vi "CreateSEQ.vi"() -> (3 "FPGA out":refnum<queue>, 5 "created new?":bool)   [LabVIEW 2019, in "FPGA.lvlib"]
uses:
  FPGA.lvlib
  FPGA.ctl
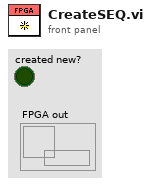
[diagram p1: front panel]
types:
  T1 = typedef "FPGA.lvlib/FPGA.ctl" = cluster{"Start freq. [Hz]":dbl, "Sweep duration [s]":dbl, "Freq. step [Hz]":dbl, "DAC Sample Rate":dbl, "ADC Sample Rate":dbl, "CMD port":u16, "DFAST port":u16, "CMD ID":refnum<k16>, "DFAST ID":refnum<k16>, "CMD error out":errorcluster, "FPGA IP":string, "DFAST error out ":errorcluster, "Stop freq. [Hz]":dbl, "Discrete sweep":bool, "Initial NCO":u32, "Difference NCO":i32, "step NCO":i64, "Final NCO":u32, "clocks for step":u32, "demodulation":bool, "NCO Phase Precision":u32, "NCO Sample Rate":dbl, "Time for step [s]":dbl, "NCO freq. resolution":dbl, "Sweep speed [Hz/s]":dbl, "Connected":bool, "Slew Rate [V/us]":dbl, "Parameters_ok":bool, "Amplitude [mVpp]":dbl, "Scale Factor":fxp<+,16,0>, "Acquiring":bool, "DAC-ADC Latency":u16, "Digital Gain":i32, "Number of steps":i32, "Averaging preferred":bool, "Filter Order":u32, "Settling":enum16{"99%", "99,9%"}}
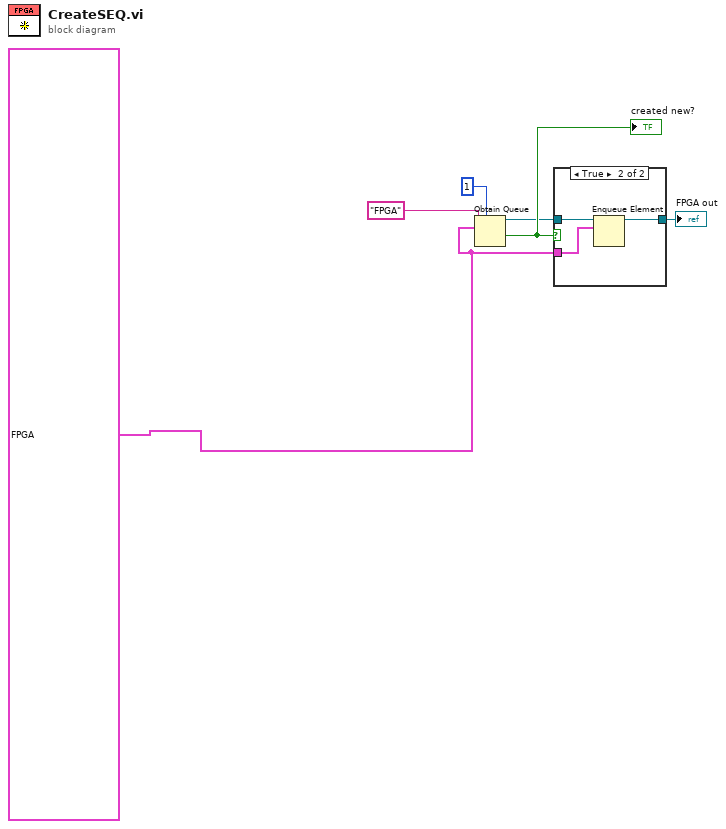
[diagram p0: block diagram]
diagram:
  w1 = T1 {"Start freq. [Hz]"=10.0, "Sweep duration [s]"=0.1, "Freq. step [Hz]"=0.1, "DAC Sample Rate"=1388888.8888, "ADC Sample Rate"=50000000.0, "CMD port"=2047, "DFAST port"=2048, "CMD ID"=refnum, "DFAST ID"=refnum, "CMD error out"={"status"=FALSE, "code"=0, "source"=""}, "FPGA IP"="192.168.1.12", "DFAST error out "={"status"=FALSE, "code"=0, "source"=""}, "Stop freq. [Hz]"=0.0, "Discrete sweep"=FALSE, "Initial NCO"=10, "Difference NCO"=0, "step NCO"=0, "Final NCO"=0, "clocks for step"=0, "demodulation"=FALSE, "NCO Phase Precision"=32, "NCO Sample Rate"=50000000.0, "Time for step [s]"=0.1, "NCO freq. resolution"=32.0, "Sweep speed [Hz/s]"=0.1, "Connected"=FALSE, "Slew Rate [V/us]"=0.8, "Parameters_ok"=FALSE, "Amplitude [mVpp]"=10.0, "Scale Factor"=0.999969482421875, "Acquiring"=FALSE, "DAC-ADC Latency"=1, "Digital Gain"=0, "Number of steps"=1, "Averaging preferred"=FALSE, "Filter Order"=1, "Settling"=enum."99,9%"} ("FPGA CLUSTER")
  n1 = Obtain Queue(max queue size (-1, unlimited)=1, name (unnamed)="FPGA" ("FPGA Name"), element data type=w1) -> (queue out=w5:refnum<queue>, created new?=w6:bool)  [unwired: 2 in, 1 out]
  "created new?" <- w6
  n2 = case shown="True" w6 {
    tunnel: w5 -> [w7 w10]
    tunnel: w1 -> [_ w9]
    tunnel: [w7 w8] -> w2
    frame False {
    }
    frame True {
      n3 = Enqueue Element(queue=w10, element=w9) -> (queue out=w8:refnum<queue>)  [unwired: 2 in, 2 out]
    }
  }
  "FPGA out" <- w2
